vi "Measurement UI.vi"() -> ()   [LabVIEW 2024, in "NIDCPowerPPS.lvlib"]
uses:
  NIDCPowerPPS.lvlib
panel:
  out "Measured Power (W)":dbl format="%#_13g"
  out "In Compliance":bool
  out "Current Measurement (A)":dbl format="%#_13g"
  out "Voltage Measurement (V)":dbl format="%#_13g"
  in  "Source Delay (s)":dbl=0.1 format="%#_13g"
  in  "Current Limit Range (A)":dbl=1.0 format="%#_13g"
  in  "Current Limit (A)":dbl=0.1 format="%#_13g"
  in  "Voltage Level Range (V)":dbl=6.0 format="%#_13g"
  in  "Voltage Level (V)":dbl=2.0 format="%#_13g"
  in  "Pin Name":string(combo)="Pin1"
  # "Input"
  # "Output"
  # "Pin Settings"
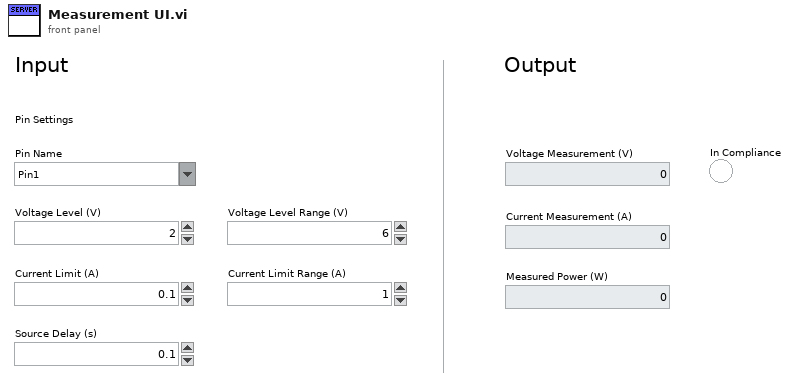
[diagram p1: front panel]
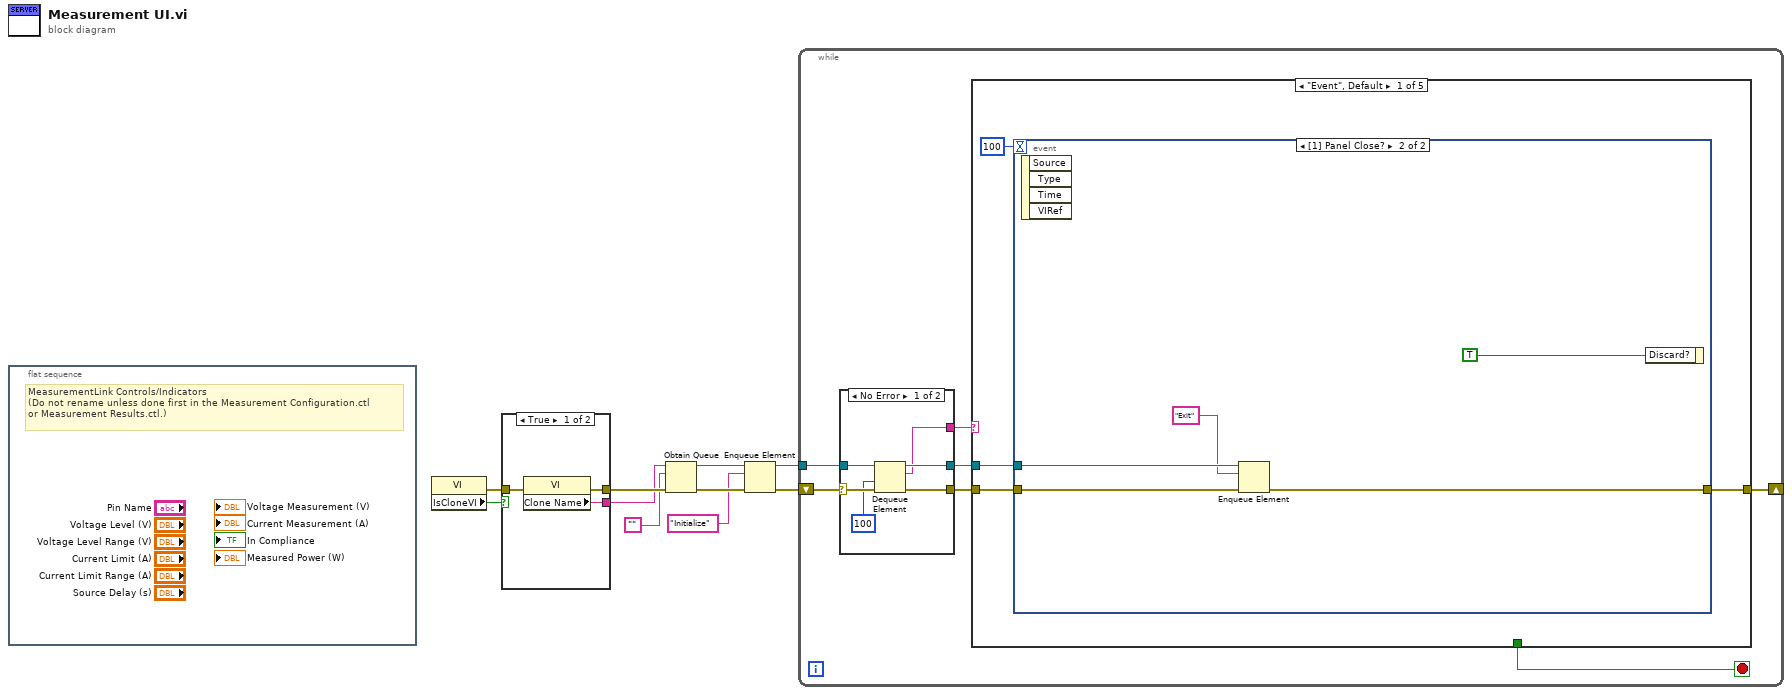
[diagram p0: block diagram]
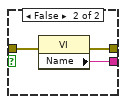
[diagram p2: hidden frame]
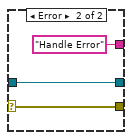
[diagram p3: hidden frame]
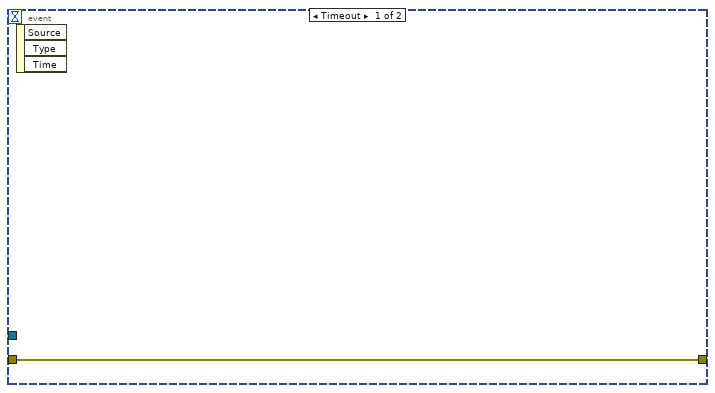
[diagram p4: hidden frame]
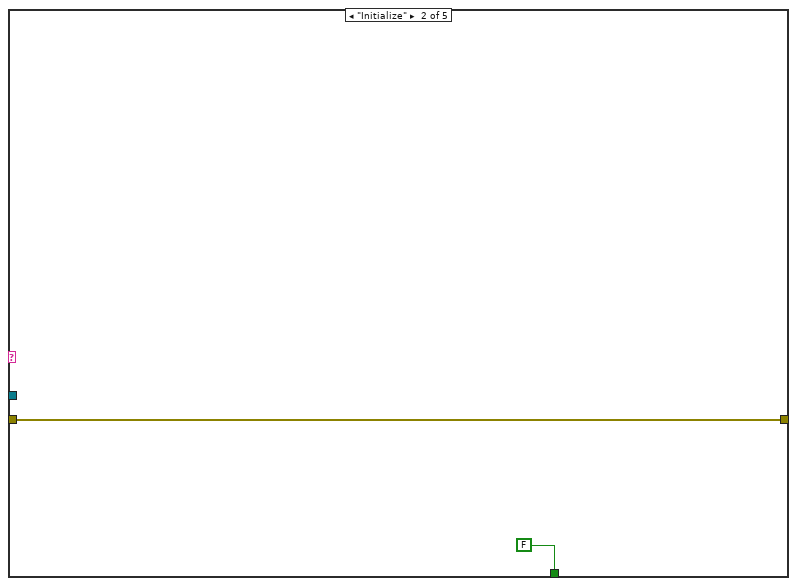
[diagram p5: hidden frame]
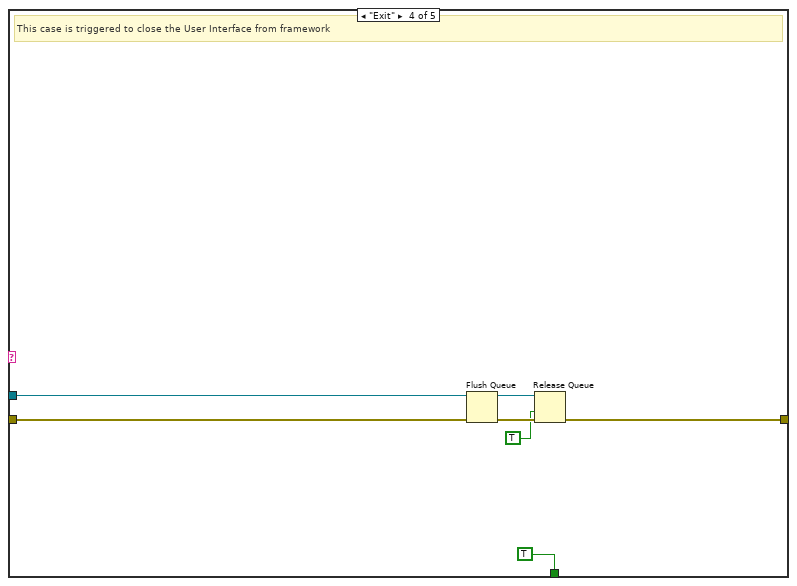
[diagram p7: hidden frame]
diagram:
  n1 = flat-sequence {
    frame #0 {
      # "MeasurementLink Controls/Indicators\n(Do not rename unless done first in the Measurement Configuration.ctl\nor Measurement Results.ctl.)"
    }
  }
  n2 = property class="VI"() -> (error out=w1:errorcluster, "IsCloneVI"=w2:bool)  [unwired: 2 in, 1 out]
  n3 = case shown="True" w2 {
    tunnel: [w13 w16] -> w10
    tunnel: [w12 w15] -> w9
    tunnel: w1 -> [w11 w14]
    frame True {
      n4 = property class="VI"(error in=w11) -> (error out=w13:errorcluster, "Clone Name"=w12:string)  [unwired: 1 in, 1 out]
    }
    frame False {
      n5 = property class="VI"(error in=w14) -> (error out=w16:errorcluster, "Name"=w15:string)  [unwired: 1 in, 1 out]
    }
  }
  n6 = Obtain Queue(name (unnamed)=w9, element data type="", error in (no error)=w10) -> (queue out=w6:refnum<queue>, error out=w8:errorcluster)  [unwired: 2 in, 1 out]
  n7 = Enqueue Element(queue=w6, element="Initialize", error in (no error)=w8) -> (queue out=w5:refnum<queue>, error out=w7:errorcluster)  [unwired: 1 in, 1 out]
  n8 = while {
    shift-right: [w18] -> _
    shift-left: w7 -> [w23]
    tunnel: w5 -> [w21]
    stop <- w17 stop-if-true
    n9 = case shown="No Error" w23 {
      selector: w23 -> [w29 w32]
      tunnel: [w28 w32] -> w22
      tunnel: w21 -> [w27 w31]
      tunnel: [w26 w31] -> w20
      tunnel: [w25 "Handle Error"] -> w19
      frame No Error {
        n10 = Dequeue Element(queue=w27, timeout in ms (-1)=100, error in (no error)=w29) -> (queue out=w26:refnum<queue>, element=w25:string, error out=w28:errorcluster)  [unwired: 1 out]
      }
      frame Error {
      }
    }
    n11 = case shown="\"Event\", Default" w19 {
      tunnel: w22 -> [w35 w44 w45 w52 w53]
      tunnel: w20 -> [w33 _ _ w50 _]
      tunnel: [w36 w44 w45 w47 w53] -> w18
      tunnel: [_ FALSE _ TRUE _] -> w17
      frame "Event", Default {
        n12 = event shown="[1] Panel Close?" {
          selector: _ -> [_ _]
          dyn-events: _ -> [_ _]
          timeout: 100 -> [_ _]
          tunnel: [w37 w40] -> w36
          tunnel: w35 -> [w37 w41]
          tunnel: w33 -> [_ w39]
          event Timeout {
            n13 = event-data() -> ()  [unwired: 1 in, 3 out]
          }
          event Panel Close? {
            n14 = event-data() -> ()  [unwired: 1 in, 4 out]
            n15 = Enqueue Element(queue=w39, element="Exit", error in (no error)=w41) -> (error out=w40:errorcluster)  [unwired: 1 in, 2 out]
            n16 = event-data("Discard?"=TRUE) -> ()  [unwired: 1 in, 1 out]
          }
        }
      }
      frame "Initialize" {
      }
      frame "Post UI Update" {
        # "This case will be triggered, after framework updates the User interface with result values."
      }
      frame "Exit" {
        # "This case is triggered to close the User Interface from framework"
        n17 = Flush Queue(queue=w50, error in (no error)=w52) -> (queue out=w49:refnum<queue>, error out=w48:errorcluster)  [unwired: 1 out]
        n18 = Release Queue(queue=w49, force destroy? (F)=TRUE, error in (no error)=w48) -> (error out=w47:errorcluster)  [unwired: 2 out]
      }
      frame "Handle Error" {
      }
    }
  }
